vi "SetScanEnc.vi"(8 "错误输入（无错误）":errorcluster, 10 "扫查编码器":u32) -> (0 "错误输出":errorcluster)   [LabVIEW 2014]
uses:
  X86Dll/ZXUTConfigMgr.dll
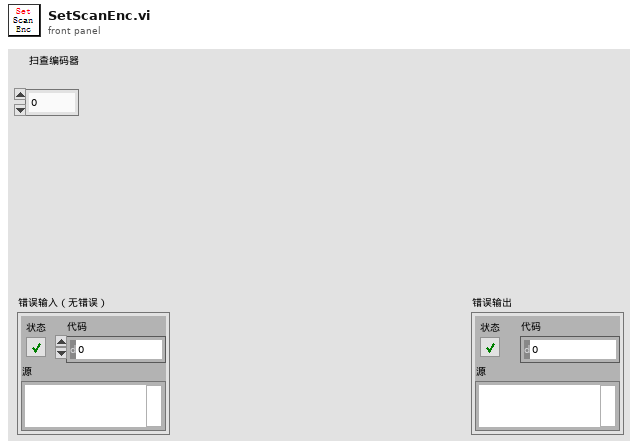
[diagram p1: front panel]
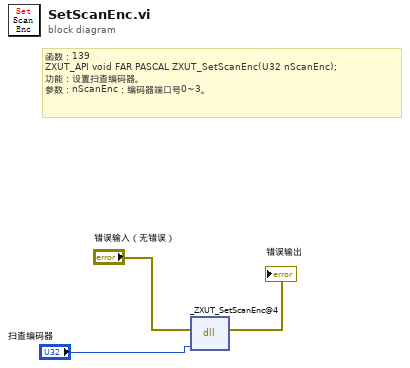
[diagram p0: block diagram]
diagram:
  # "函数：139\nZXUT_API void\tFAR PASCAL ZXUT_SetScanEnc(U32 nScanEnc);\n功能：设置扫查编码器。\n参数：nScanEnc：编码器端口号0~3。"
  n1 = dll-call lib="D:/Software/Utrasonic on-line monitoring/X86Dll/ZXUTConfigMgr.dll" fn="_ZXUT_SetScanEnc@4"(error in="错误输入（无错误）", "nScanEnc"="扫查编码器") -> (error out=→"错误输出":errorcluster)  [unwired: 4 in, 1 out]
